vi "SetHightAngle.vi"(8 "error in (no error)":errorcluster, 9 "Wrist (degrees)":dbl, 10 "Main arm(degrees)":dbl, 11 "Elevator Concrete in":refnum<class "Elevator Concrete.lvclass">) -> (0 "error out":errorcluster, 3 "Elevator Concrete out":refnum<class "Elevator Concrete.lvclass">)   [LabVIEW 2018, in "Elevator.lvlib" / "Elevator Concrete.lvclass"]
uses:
  Elevator Concrete.lvclass
  C:/Users/Public/Documents/2019DeepSpace/Classes/Elevator/Elevator.lvclass
  <vilib>/Rock Robotics/WPI/ThirdParty/Phoenix-LabVIEW/Motor Controller/Controls/CTRE_Phoenix_MotorControl_ControlMode.ctl
  Elevator Concrete.lvclass/Elevator Concrete.ctl
  Elevator.lvclass
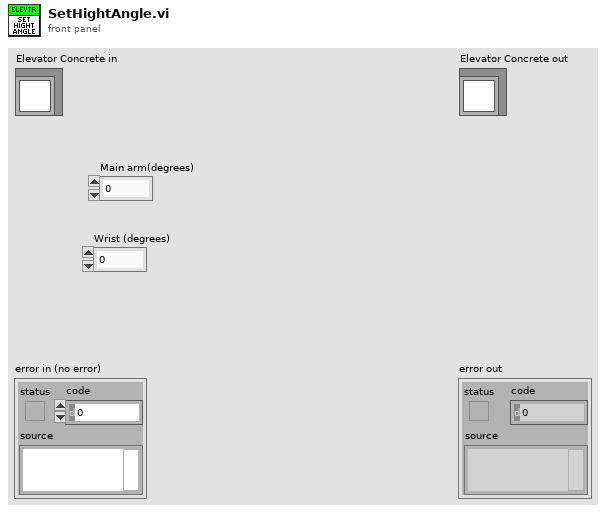
[diagram p1: front panel]
types:
  T1 = typedef "CTRE_Phoenix_MotorControl_ControlMode.ctl" = u16
  T2 = typedef "Elevator.lvlib/Elevator.lvclass/Elevator Constants.ctl" = cluster{"Arm Motion Magic Max Velocity":u32, "Arm Motion Magic Max Acceleration":u32, "Wrist Motion Magic Max Velocity":u32, "Wrist Motion Magic Max Acceleration":u32, "Arm Gear Ratio":dbl, "Wrist Gear Ratio":dbl, "Arm Encoder ABS Value":i32, "Wrist Encoder ABS Value":i32}
  T3 = typedef "WPI_MotorControlDeviceRef.ctl" = cluster{"DeviceStatus":errorcluster, "Type":T4, "PWM":cluster{"PWM Channel":T5, "DeadBand":T6}, "CAN":cluster{"Device Number":u8, "SetOutput VI Ref":variant, "GetOutput VI Ref":variant, "Enable VI Ref":variant, "Disable VI Ref":variant, "Data":variant}, "Invert":bool, "DIO PWM":cluster{"PWM \"Enable\" Channel":T5, "DIOChannel":T7, "PWM Rate":dbl}}
  T4 = typedef "WPI_MotorControlType.ctl" = enum16{"PWM", "CAN", "DIO PWM"}
  T5 = typedef "FPGA_DIOPWMChannel.ctl" = enum8{"PWM 0", "PWM 1", "PWM 2", "PWM 3", "PWM 4", "PWM 5", "PWM 6", "PWM 7", "PWM 8", "PWM 9", "PWM MXP 0", "PWM MXP 1", "PWM MXP 2", "PWM MXP 3", "PWM MXP 4", "PWM MXP 5", "PWM MXP 6", "PWM MXP 7", "PWM MXP 8", "PWM MXP 9", "Invalid"}
  T6 = typedef "WPI_PWMDeadband.ctl" = cluster{"Name":string, "maxPositivePwm":i32, "minPositivePwm":i32, "centerPwm":i32, "maxNegativePwm":i32, "minNegativePwm":i32, "angularRange":u16}
  T7 = typedef "FPGA_DIOChannel.ctl" = enum8{"DIO 0", "DIO 1", "DIO 2", "DIO 3", "DIO 4", "DIO 5", "DIO 6", "DIO 7", "DIO 8", "DIO 9", "DIO MXP 0", "DIO MXP 1", "DIO MXP 2", "DIO MXP 3", "DIO MXP 4", "DIO MXP 5", "DIO MXP 6", "DIO MXP 7", "DIO MXP 8", "DIO MXP 9", "DIO MXP 10", "DIO MXP 11", "DIO MXP 12", "DIO MXP 13", "DIO MXP 14", "DIO MXP 15", "SPI Port CS1", "SPI Port CS2", "SPI Port CS3", "SPI Port MISO", "SPI Port MOSI", "Invalid"}
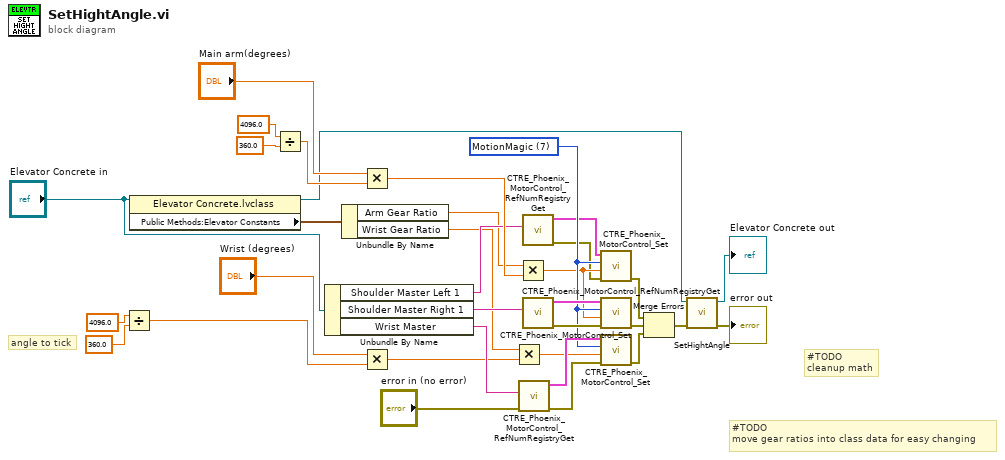
[diagram p0: block diagram]
diagram:
  w15 = T1 7 items=["PercentOutput"=0, "Position"=1, "Velocity"=2, "Current"=3, "Follower"=5, "MotionProfile"=6, "MotionMagic"=7, "MotionProfileArc"=10, "Disabled"=15] ("Control Mode")
  # "#TODO\nmove gear ratios into class data for easy changing"
  # "#TODO\ncleanup math"
  # "angle to tick"
  n1 = Divide(x=4096.0, y=360.0) -> (x/y=w5:dbl)
  n2 = property class="Elevator Concrete.lvclass"(reference="Elevator Concrete in") -> (reference out=w4:refnum<class "Elevator Concrete.lvclass">, "Public Methods:Elevator Constants"=w3:T2)  [unwired: 1 in, 1 out]
  n3 = Divide(x=4096.0, y=360.0) -> (x/y=w19:dbl)
  n4 = Unbundle By Name("Elevator Concrete in") -> ("Shoulder Master Left 1"=w16:string, "Shoulder Master Right 1"=w29:string, "Wrist Master"=w26:string)
  n5 = Unbundle By Name(w3) -> ("Arm Gear Ratio"=w2:dbl, "Wrist Gear Ratio"=w1:dbl)
  n6 = Multiply(x="Main arm(degrees)", y=w19) -> (x*y=w18:dbl)
  n7 = Multiply(x="Wrist (degrees)", y=w5) -> (x*y=w7:dbl)
  n8 = Multiply(x=w1, y=w7) -> (x*y=w17:dbl)
  n9 = Multiply(x=w2, y=w18) -> (x*y=w14:dbl)
  n10 = call <vilib>:"CTRE_Phoenix_MotorControl_RefNumRegistryGet.vi"("error in (no error)"="error in (no error)", "refnum name"=w26) -> ("error out"=w28:errorcluster, "PhoenixMotorControlDevRef"=w27:T3)  [unwired: 8 in]
  n11 = call <vilib>:"CTRE_Phoenix_MotorControl_RefNumRegistryGet.vi"("refnum name"=w16) -> ("error out"=w13:errorcluster, "PhoenixMotorControlDevRef"=w12:T3)  [unwired: 9 in]
  n12 = call <vilib>:"CTRE_Phoenix_MotorControl_RefNumRegistryGet.vi"("refnum name"=w29) -> ("error out"=w31:errorcluster, "PhoenixMotorControlDevRef"=w30:T3)  [unwired: 9 in]
  n13 = call <vilib>:"CTRE_Phoenix_MotorControl_Set.vi"("error in (no error)"=w13, "Output"=w14, "Control Mode"=w15, "PhoenixMotorControlDevRef"=w12) -> ("error out"=w8:errorcluster)  [unwired: 6 in, 1 out]
  n14 = call <vilib>:"CTRE_Phoenix_MotorControl_Set.vi"("error in (no error)"=w31, "Output"=w14, "Control Mode"=w15, "PhoenixMotorControlDevRef"=w30) -> ("error out"=w23:errorcluster)  [unwired: 6 in, 1 out]
  n15 = call <vilib>:"CTRE_Phoenix_MotorControl_Set.vi"("error in (no error)"=w28, "Output"=w17, "Control Mode"=w15, "PhoenixMotorControlDevRef"=w27) -> ("error out"=w25:errorcluster)  [unwired: 6 in, 1 out]
  n16 = Merge Errors(w8, w23, w25) -> (w22:errorcluster)
  n17 = call-parent "SetHightAngle.vi"("error in (no error)"=w22, "Elevator in"=w4) -> ("error out"=→"error out":errorcluster, "Elevator out"=→"Elevator Concrete out":refnum<class "Elevator Concrete.lvclass">)  [unwired: 8 in]
